vi "Button_Customize.vi"() -> ()   [LabVIEW 2013]
panel:
  in  "TEST-Button":bool
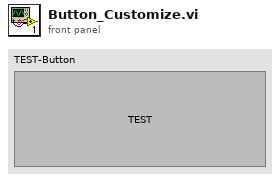
[diagram p1: front panel]
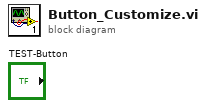
[diagram p0: block diagram]
diagram:
